vi "Generate.vi"(6 "Priority?":bool, 9 "Msg Strategy":refnum<class "Msg Strategy.lvclass">, 10 "Self Event":refnum<data-value>) -> (0 "error out":errorcluster)   [LabVIEW 2021, in "jettl.lvlib" / "Self Event.lvlib"]
uses:
  Self Event.lvlib
  Msg Strategy/Msg Strategy.lvclass
  <vilib>/event_ctls.llb/usereventprio.ctl
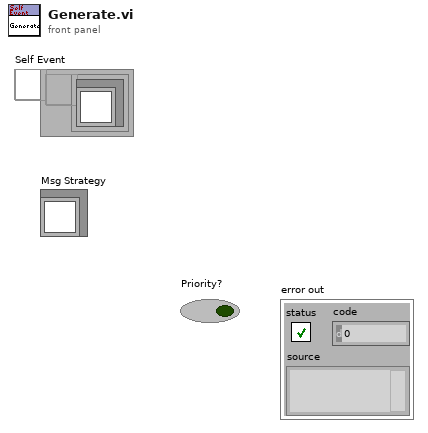
[diagram p1: front panel]
types:
  T1 = typedef "usereventprio.ctl" = enum32{"high priority", "normal priority"}
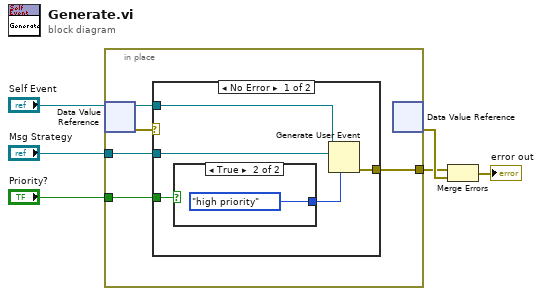
[diagram p0: block diagram]
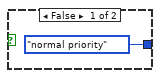
[diagram p2: hidden frame]
diagram:
  n1 = in-place {
    in-place-border: "Msg Strategy" -> [w11]
    in-place-border: [w10] -> w4
    in-place-border: "Priority?" -> [w7]
    n2 = in-place-dvr #1("Self Event") -> (w9:refnum<user-event>, w8:errorcluster)
    n3 = case shown="No Error" w8 {
      selector: w8 -> [_ w19]
      tunnel: w11 -> [w16 _]
      tunnel: [w15 w19] -> w10
      tunnel: w9 -> [w14 _]
      tunnel: w7 -> [w12 _]
      frame No Error {
        n4 = case shown="True" w12 {
          tunnel: [usereventprio."normal priority" ("priority (normal)") usereventprio."high priority" ("priority (normal)")] -> w13
          frame False {
          }
          frame True {
          }
        }
        n5 = Generate User Event(priority (normal)=w13, user event=w14, event data cluster=w16) -> (error out=w15:errorcluster)  [unwired: 1 in, 1 out]
      }
      frame Error {
      }
    }
    n6 = in-place-dvr #1() -> (w5:errorcluster)  [unwired: 1 in, 1 out]
  }
  n7 = Merge Errors(w4, w5) -> (→"error out":errorcluster)
